vi "Third Restarts by Flow Sandbox (FPGA).vi"() -> ()   [LabVIEW 2019]
uses:
  <vilib>/eio/EIONode/EIONode.xnode
  <vilib>/rvi/eio/common/nirviEmuTemplateMethod_errors.vi
  <vilib>/rvi/FXPMathLib/FxpMul/XNode/nifxpmath_Multiplier.xnode
  <vilib>/rvi/FXPMathLib/sim/FxpSim.dll
  <vilib>/Platform/TimedLoop/XDataNode/wakeup.ctl
  <vilib>/Platform/TimedLoop/XDataNode/XDNodeRunTimeDep.lvlib
  <vilib>/Platform/TimedLoop/XDataNode/nitl_modes.ctl
  <vilib>/Platform/TimedLoop/XDataNode/timing_clust.ctl
  <vilib>/Platform/TimedLoop/XDataNode/XDataNode.xnode
  <vilib>/rvi/Analysis/measure/dc-rms/XNode/niFpgaDC-RMS.xnode
  <vilib>/rvi/DataTransferAndStorage/Container/XNode/niFpgaContainer.xnode
  <vilib>/rvi/FXPMathLib/FxpAdd/XNode/nifxpmath_Add.xnode
  <userlib>/_NI SPI IP/FPGA/Controllers/Public/Spi Master Inputs.ctl
  <vilib>/eio/EIOMethodNode/EIOMethodNode.xnode
  Controls/SPI Channels.ctl
  <vilib>/rvi/FIFO/Fifo_Resource/niFpgaFifoEmulationRefIn.vi
  <vilib>/rvi/interface/RandomDataEmulation/nirviRandomDataFpgaReadWriteTemplate.vi
  <vilib>/rvi/FXPMathLib/basic elements/FxpIntAccumulator/simVIs/DllFxpIntAccumulator_sub.vi
  <vilib>/rvi/FXPMathLib/basic elements/FxpIntAccumulator/XNode/nifxpmath_IntAccumulator.xnode
  <vilib>/rvi/FXPMathLib/FxpSqrt/XNode/nifxpmath_Sqrt.xnode
  <vilib>/rvi/Analysis/common/codeGenErrors/XNode/niFpgaXNodeCodeGenErrorHandle.vi
  <vilib>/rvi/FXPMathLib/FxpSqrt/simVIs/DllSqrtTemp_sub.vi
  <vilib>/fxp/LVFixedPointOverflowPolicyTypeDef.ctl
  <vilib>/rvi/FXPMathLib/FxpSqrt/subVIs/nifxpmath_Sqrt_SimConfig.ctl
  <vilib>/rvi/FXPMathLib/basic elements/FxpIntAccumulator/subVIs/nifxpmath_IntAccumulator_SimConfig.ctl
  <vilib>/rvi/FXPMathLib/FxpSub/XNode/nifxpmath_Sub.xnode
  <userlib>/_NI SPI IP/FPGA/Controllers/Public/Transfer Settings.ctl
panel:
  in  "Trigger":bool
  in  "Reset Restarts":bool
  in  "AI24-31 Data to Write":u64 format="%.0x"
  out "AI24-31":fxp<+/-,28,17>[](array[numeric])
  out "Read Data 2":u64 format="%.0x"
  in  "AI24-31 Settings":T1 {"Direction Change Bit" max=64 step=1; "Transfer Length (bits)" min=1 max=64 step=1}
  out "AI16-23":fxp<+/-,28,17>[](array[numeric])
  in  "AI16-23 Data to Write":u64 format="%.0x"
  out "Read Data":u64 format="%.0x"
  in  "AI16-23 Settings":T1 {"Direction Change Bit" max=64 step=1; "Transfer Length (bits)" min=1 max=64 step=1}
  in  "AO0":fxp<+/-,20,5>
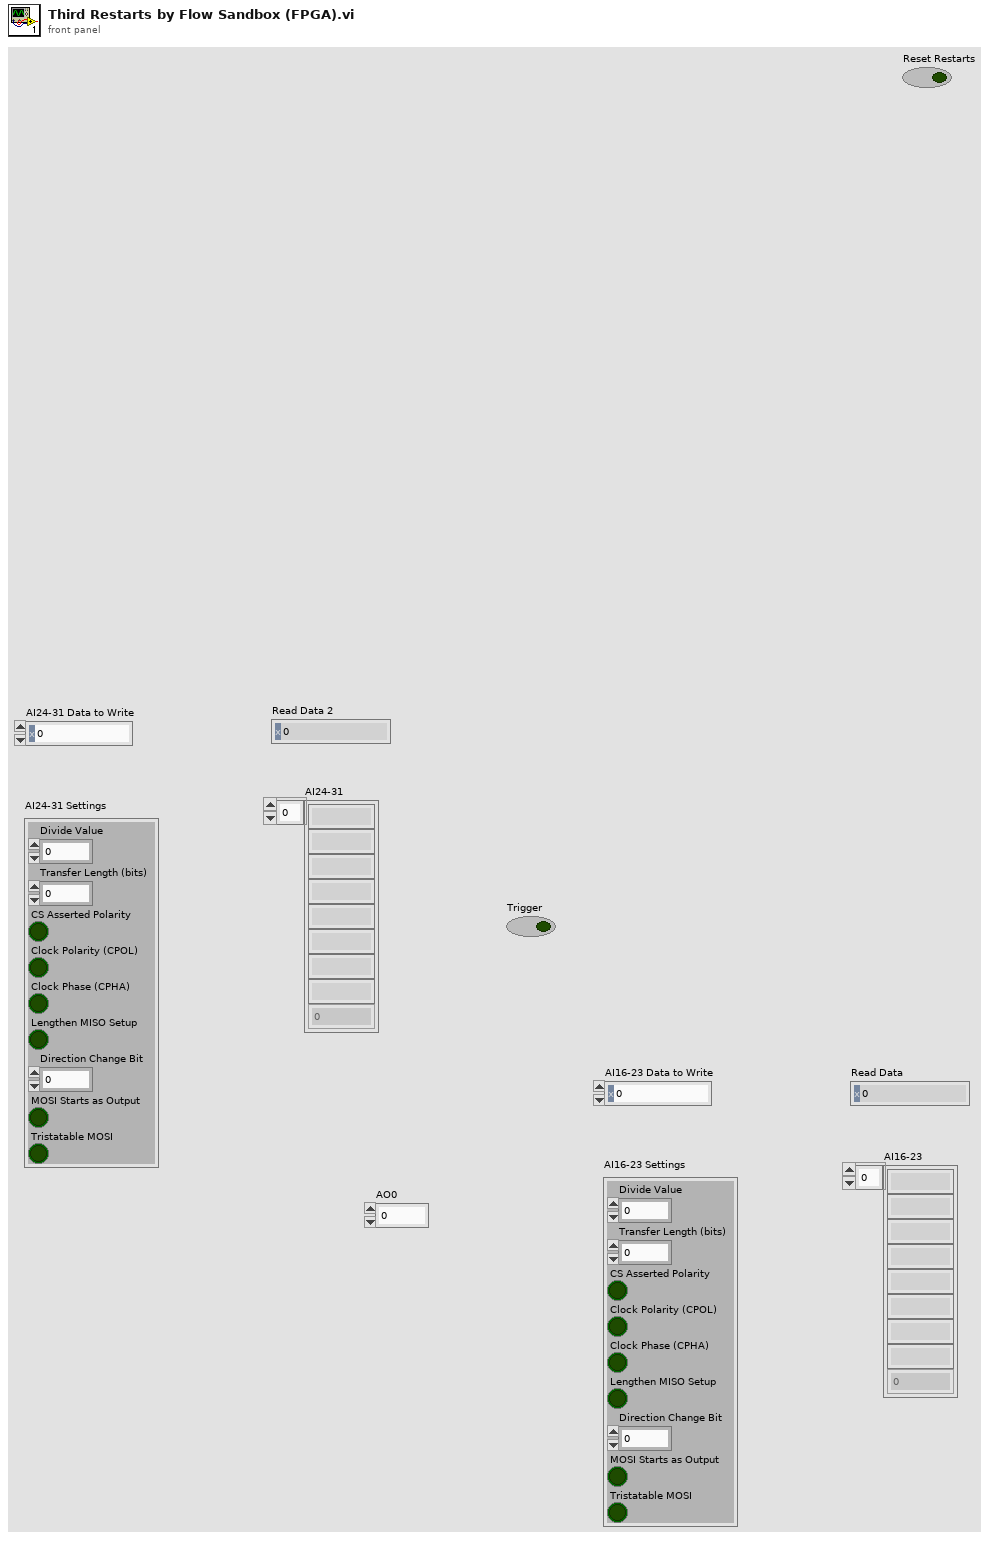
[diagram p1: front panel]
types:
  T1 = typedef "DIO SPI FPGA.lvlib/Transfer Settings.ctl" = cluster{"Divide Value":u8, "Transfer Length (bits)":u8, "CS Asserted Polarity":bool, "Clock Polarity (CPOL)":bool, "Clock Phase (CPHA)":bool, "Lengthen MISO Setup":bool, "Direction Change Bit":u8, "MOSI Starts as Output":bool, "Tristatable MOSI":bool}
  T2 = typedef "SPI Channels.ctl" = cluster{"CS":refnum<k21>, "CLK":refnum<k21>, "MOSI":refnum<k21>, "MISO":refnum<k21>}
  T3 = typedef "XDNodeRunTimeDep.lvlib/timing_clust.ctl" = cluster{"Expected End [f-1]":u64, "Actual End [f-1]":u64, "Finished Late? [f-1]":bool, "Expected End [i-1]":u64, "Actual End [i-1]":u64, "Finished Late? [i-1]":bool, "Expected Start [i]":u64, "Actual Start [i]":u64, "Expected Start [f]":u64, "Actual Start [f]":u64, "Source Name":string, "Structure Name":string, "Period":i64, "Deadline":i64, "Offset":i64, "Start":i64, "Priority":i32, "Timeout":i32, "Mode":T4, "Wakeup Reason":T5, "Error":errorcluster, "Source Type":string, "Secondary Source Type":string, "Global End Time":u64, "Global Start Time":u64, "Frame Duration":u64, "Iteration Duration":u64, "Assigned CPU":i32, "I/O Scan Engine Mode":u32}
  T4 = typedef "XDNodeRunTimeDep.lvlib/nitl_modes.ctl" = enum32{"No Change", "Process missed periods, maintain original phase", "Discard missed periods, maintain original phase", "Process missed periods, ignore original phase", "Discard missed periods, ignore original phase"}
  T5 = typedef "XDNodeRunTimeDep.lvlib/wakeup.ctl" = enum32{"Normal", "Aborted", "Asynchronous wakeup", "Timing source error", "Timed loop error", "Timeout"}
  T6 = typedef "DIO SPI FPGA.lvlib/Spi Master Inputs.ctl" = cluster{"MISO":bool}
  T7 = typedef "DIO SPI FPGA.lvlib/Spi Master Outputs.ctl" = cluster{"Chip Select":bool, "Clock":bool, "MOSI":bool, "MOSI OE":bool}
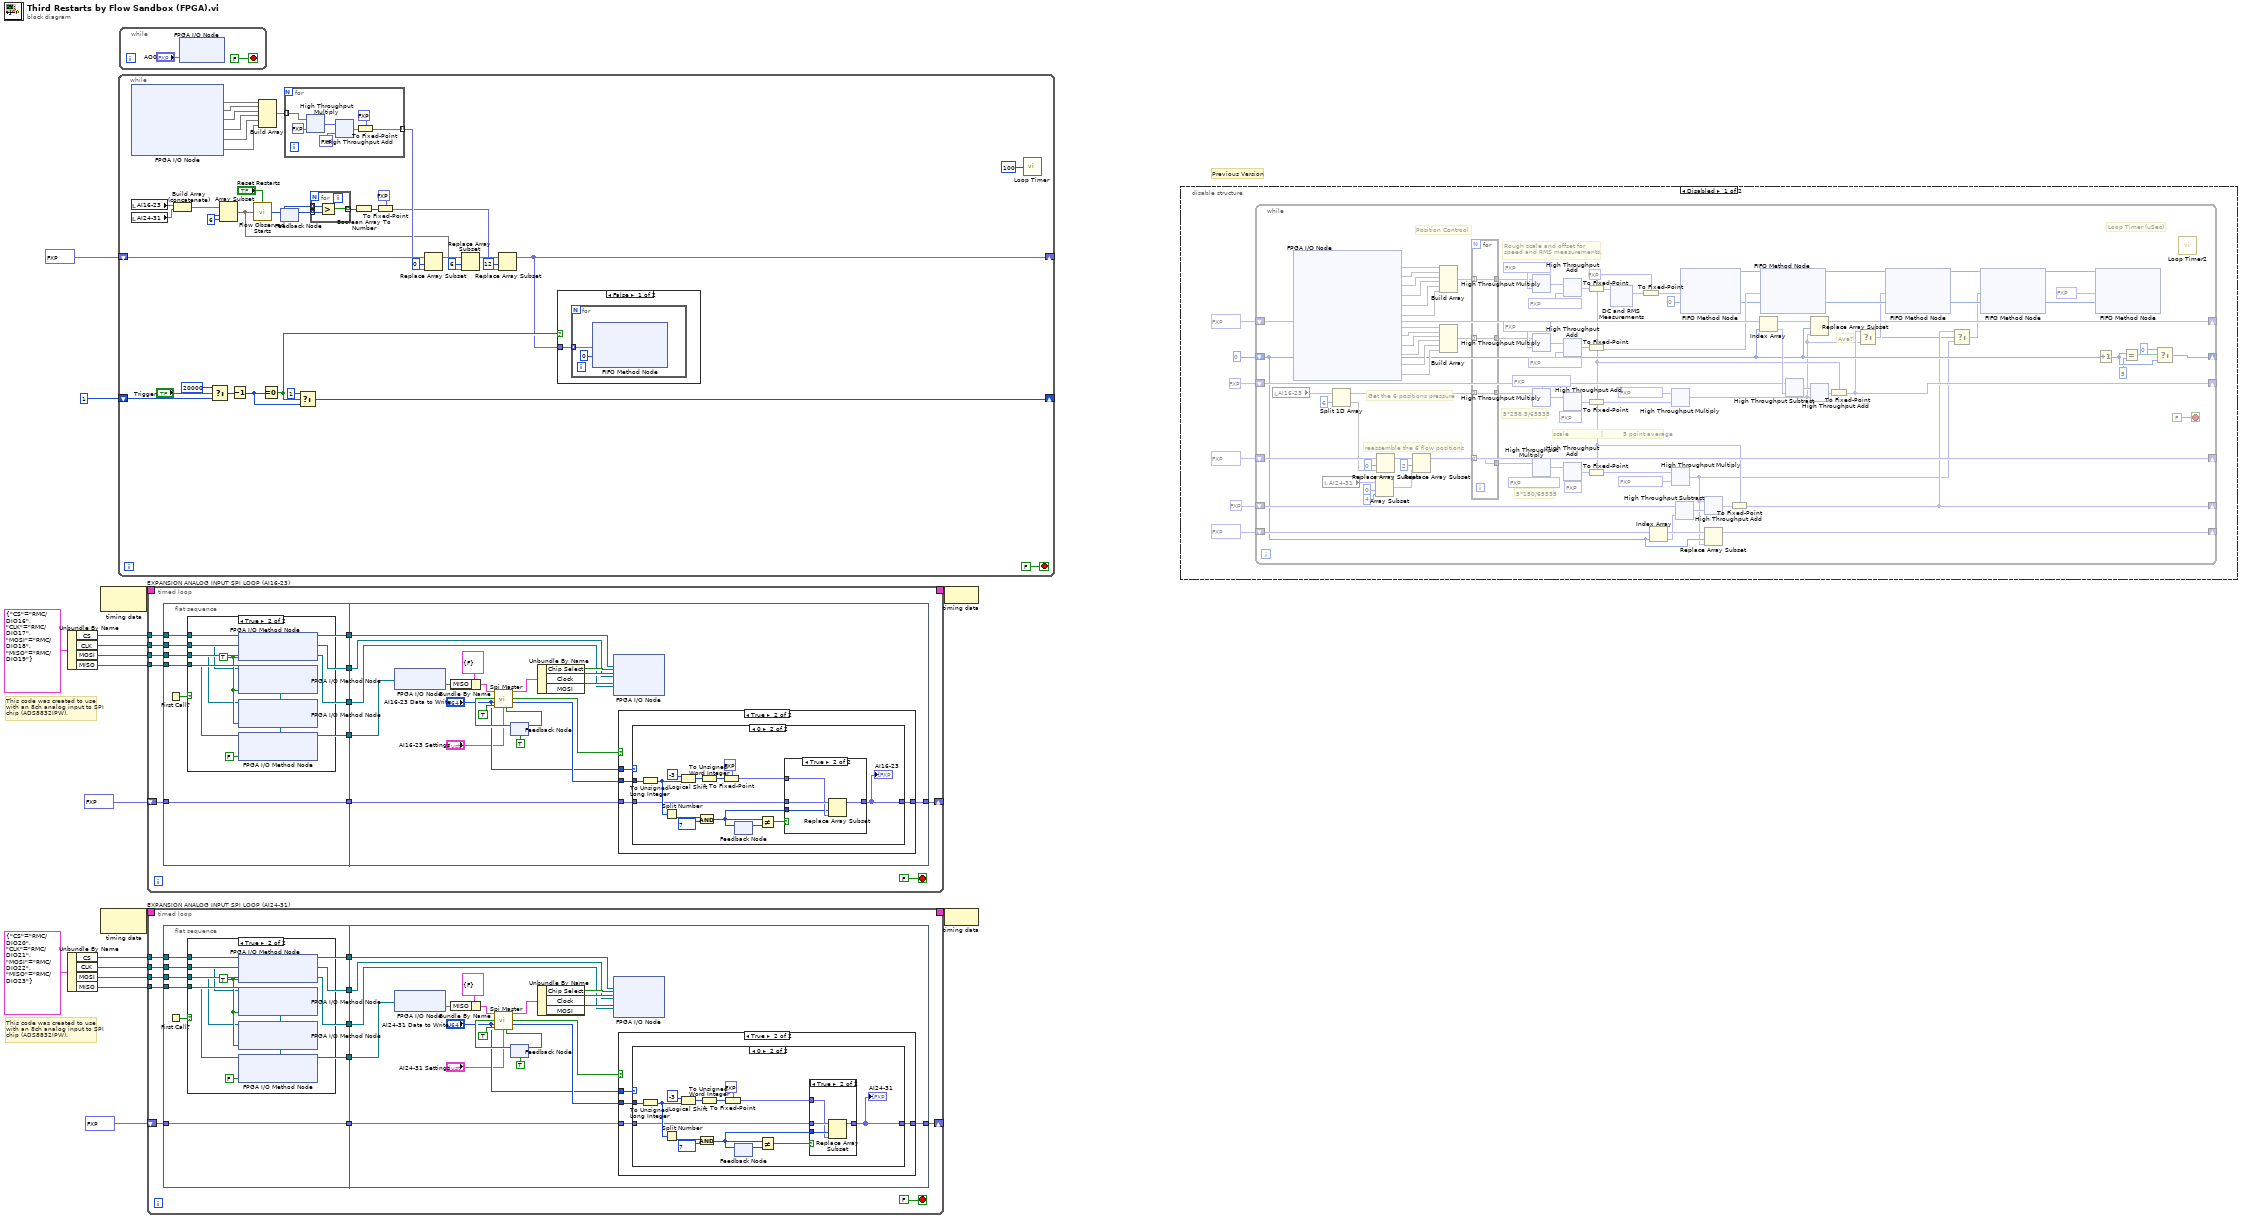
[diagram p0: block diagram]
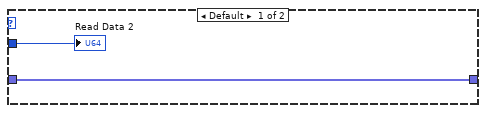
[diagram p6: hidden frame]
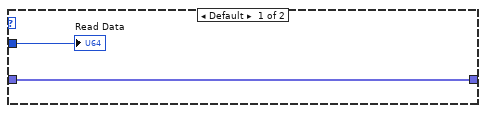
[diagram p10: hidden frame]
diagram:
  # "Previous Version"
  # "This code was created to use\nwith an 8ch analog input to SPI\nchip (ADS8832IPW)."
  # "This code was created to use\nwith an 8ch analog input to SPI\nchip (ADS8832IPW)."
  n1 = Unbundle By Name(T2 {"CS"="RMC/DIO16", "CLK"="RMC/DIO17", "MOSI"="RMC/DIO18", "MISO"="RMC/DIO19"} ("SPI Channels")) -> ("CS"=w12:refnum<k21>, "CLK"=w13:refnum<k21>, "MOSI"=w14:refnum<k21>, "MISO"=w15:refnum<k21>)
  n2 = Unbundle By Name(T2 {"CS"="RMC/DIO20", "CLK"="RMC/DIO21", "MOSI"="RMC/DIO22", "MISO"="RMC/DIO23"} ("SPI Channels")) -> ("CS"=w4:refnum<k21>, "CLK"=w5:refnum<k21>, "MOSI"=w6:refnum<k21>, "MISO"=w7:refnum<k21>)
  n3 = node-c288() -> (w18:T3)  [unwired: 1 in]
  n4 = node-c288() -> (w10:T3)  [unwired: 1 in]
  n5 = while {
    shift-right: [w36] -> _
    shift-left: i16 1 -> [w41]
    shift-right: [w19] -> _
    shift-left: fxp<+/-,28,17>[] [0.0, 0.0, 0.0, 0.0, 0.0, 0.0, 0.0, 0.0, 0.0, 0.0, 0.0, 0.0, 0.0] -> [w29]
    stop <- FALSE stop-if-true
    w44 = 6 ("length")
    n6 = xnode "FPGA I/O Node"() -> ("Speed_Current_1 (AI0)"=w46, "Speed_Current_2 (AI1)"=w51, "Speed_Current_3 (AI2)"=w50, "Speed_Current_4 (AI3)"=w49, "Speed_Current_5 (AI4)"=w48, "Speed_Current_6 (AI5)"=w47)  [unwired: 6 in, 6 out]
    n7 = local read "AI16-23"() -> (w54:fxp<+/-,28,17>[])
    n8 = local read "AI24-31"() -> (w55:fxp<+/-,28,17>[])
    n9 = Build Array (concatenate)(w54, w55) -> (w45:fxp<+/-,28,17>[])
    n10 = Select(t=i16 20000, s="Trigger", f=w41) -> (s? t:f=w39:i16)
    n11 = Array Subset(array=w45, index=w44, length=w44) -> (w25:fxp<+/-,28,17>[])
    n12 = Decrement(x=w39) -> (x-1=w38:i16)
    n13 = call "Flow Observed Starts.vi"("Reset Starts"="Reset Restarts", "Flows"=w25) -> ("Observed Starts"=w34:u32[])  [unwired: 13 in]
    n14 = Build Array(w46, w51, w50, w49, w48, w47) -> (w30:void[])
    n15 = Equal To 0?(x=w38) -> (x = 0?=w20:bool)
    n16 = feedback-in #1(w34) -> ()
    n17 = feedback #1(w34) -> (w35:u32[])
    n18 = for {
      tunnel: w30 -> [w60] mode=indexing
      tunnel: [w59] -> w26 mode=indexing
      n19 = xnode ("High Throughput Multiply")("x"=w60, "y"=fxp<+,5,5> 24.0 ("Current Scale")) -> ("x*y"=w63:fxp<+/-,29,10>)
      n20 = xnode ("High Throughput Add")("x"=w63, "y"=fxp<+/-,7,7> -60.0 ("Current Offset")) -> ("x+y"=w65:fxp<+/-,30,11>)
      n21 = To Fixed-Point(fixed-point type=fxp<+/-,28,17> 0.0 ("out"), number=w65) -> (fixed-point=w59:fxp<+/-,28,17>)
    }
    n22 = Select(t=i16 1, s=w20, f=w38) -> (s? t:f=w36:i16)
    n23 = for {
      tunnel: w35 -> [w67] mode=indexing
      tunnel: w34 -> [w68] mode=indexing
      tunnel: [w66] -> w33 mode=indexing
      n24 = Greater?(x=w68, y=w67) -> (0:w66:bool)
    }
    n25 = Boolean Array To Number(Boolean array=w33) -> (number=w31:u8)
    n26 = To Fixed-Point(fixed-point type=fxp<+/-,28,17> 0.0 ("out"), number=w31) -> (fixed-point=w24:fxp<+/-,28,17>)
    n27 = Replace Array Subset(array=w29, new element=w26, index=0) -> (w28:fxp<+/-,28,17>[])
    n28 = Replace Array Subset(array=w28, new element=w25, index=6) -> (w27:fxp<+/-,28,17>[])
    n29 = Replace Array Subset(array=w27, new element=w24, index=12) -> (w19:fxp<+/-,28,17>[])
    n30 = case shown="False" w20 {
      tunnel: w19 -> [w56 _]
      frame False {
        n31 = for {
          tunnel: w56 -> [w57] mode=indexing
          n32 = xnode ("FIFO Method Node")("Element"=w57, "Timeout"=0) -> ()  [unwired: 1 in, 2 out]
        }
      }
      frame True {
      }
    }
    n33 = call "Loop Timer"("Count(uSec)"=u32 100 ("Loop Timer (uSec)")) -> ()  [unwired: 1 out]
  }
  n34 = while {
    stop <- FALSE stop-if-true
    n35 = xnode "FPGA I/O Node"("AO0"="AO0") -> ()  [unwired: 2 in, 2 out]
  }
  n36 = timed-loop "EXPANSION ANALOG INPUT SPI LOOP (AI16-23)" {
    timing: w18 -> [_]
    timing-out: [_] -> w17
    shift-right: [w79] -> _
    shift-left: fxp<+/-,28,17>[] [0.0, 0.0, 0.0, 0.0, 0.0, 0.0, 0.0, 0.0] -> [w80]
    tunnel: w12 -> [w78]
    tunnel: w13 -> [w77]
    tunnel: w14 -> [w76]
    tunnel: w15 -> [w75]
    stop <- FALSE stop-if-true
    n37 = flat-sequence {
      tunnel: [w87] -> w81
      tunnel: w80 -> [w87]
      tunnel: w78 -> [w86]
      tunnel: w77 -> [w85]
      tunnel: w76 -> [w84]
      tunnel: w75 -> [w83]
      tunnel: [w86] -> w74
      tunnel: [w85] -> w73
      tunnel: [w84] -> w72
      tunnel: [w83] -> w71
      tunnel: w81 -> [w101]
      tunnel: [w100] -> w79
      tunnel: w74 -> [w99]
      tunnel: w73 -> [w98]
      tunnel: w72 -> [w97]
      tunnel: w71 -> [w96]
      frame #0 {
        n38 = First Call?() -> (First Call?: T/F=w88:bool)
        n39 = case shown="True" w88 {
          tunnel: w86 -> [_ w92]
          tunnel: w85 -> [_ w91]
          tunnel: w84 -> [_ w90]
          tunnel: w83 -> [_ w89]
          frame False {
          }
          frame True {
            w94 = TRUE ("Enable")
            n40 = xnode "FPGA I/O Method Node"("FPGA I/O In"=w92, "Enable"=w94) -> ()  [unwired: 1 out]
            n41 = xnode "FPGA I/O Method Node"("FPGA I/O In"=w91, "Enable"=w94) -> ()  [unwired: 1 out]
            n42 = xnode "FPGA I/O Method Node"("FPGA I/O In"=w90, "Enable"=w94) -> ()  [unwired: 1 out]
            n43 = xnode "FPGA I/O Method Node"("FPGA I/O In"=w89, "Enable"=FALSE) -> ()  [unwired: 1 out]
          }
        }
      }
      frame #1 {
        n44 = xnode "FPGA I/O Node"("FPGA I/O In"=w96) -> ("I/O Item"=w109)  [unwired: 1 out]
        n45 = Bundle By Name(cluster=T6 {"MISO"=FALSE} ("spi input"), "MISO"=w109) -> (w110:T6)
        n46 = feedback #2(TRUE ("read data valid")) -> (w106:bool)
        n47 = call <userlib>:"Spi Master.vi"("spi input"=w110, "start strobe"=w106, "data to write"="AI16-23 Data to Write", "MOSI output enable done"=TRUE, "spi transfer settings"="AI16-23 Settings") -> ("spi output"=w115:T7, "read data valid"=w102:bool, "read data"=w107:u64, "ready for input"=w103:bool)  [unwired: 7 in]
        n48 = feedback-in #2(w103) -> ()
        n49 = Unbundle By Name(w115) -> ("Chip Select"=w114:bool, "Clock"=w113:bool, "MOSI"=w112:bool)
        n50 = xnode "FPGA I/O Node"("I/O Item"=w114, "FPGA I/O In"=w99, "I/O Item"=w113, "FPGA I/O In"=w98, "I/O Item"=w112, "FPGA I/O In"=w97) -> ()  [unwired: 3 out]
        n51 = case shown="True" w102 {
          tunnel: w107 -> [_ w120]
          tunnel: "AI16-23 Data to Write" -> [_ w119]
          tunnel: w101 -> [w116 w118]
          tunnel: [w116 w117] -> w100
          frame False {
          }
          frame True {
            n52 = case shown="0" w119 {
              tunnel: w120 -> [w122 w136]
              tunnel: w118 -> [w121 w129]
              tunnel: [w121 w128] -> w117
              frame Default {
                "Read Data" <- w122
              }
              frame 0 {
                n53 = To Unsigned Long Integer(number=w136) -> (unsigned 32bit integer=w130:u32)
                n54 = Split Number(x=w130) -> (lo(x)=w134:u16)  [unwired: 1 out]
                n55 = Logical Shift(y=i16 -3, x=w130) -> (x << y=w131:u32)
                n56 = And(x=w134, y=u16 7) -> (x .and. y?=w126:u16)
                n57 = To Unsigned Word Integer(number=w131) -> (unsigned 16bit integer=w124:u16)
                n58 = To Fixed-Point(fixed-point type=fxp<+/-,28,17> 0.0 ("AI0"), number=w124) -> (fixed-point=w123:fxp<+/-,28,17>)
                n59 = feedback #3() -> (w135:u16)  [unwired: 1 in]
                n60 = feedback-in #3(w126) -> ()
                n61 = Not Equal?(x=w126, y=w135) -> (x != y?=w127:bool)
                n62 = case shown="True" w127 {
                  tunnel: w129 -> [w137 w141]
                  tunnel: [w137 w140] -> w128
                  tunnel: w126 -> [_ w138]
                  tunnel: w123 -> [_ w139]
                  frame False {
                  }
                  frame True {
                    n63 = Replace Array Subset(array=w141, new element=w139, index=w138) -> (w140:fxp<+/-,28,17>[])
                  }
                }
                "AI16-23" <- w128
              }
            }
          }
        }
      }
    }
  }
  n64 = timed-loop "EXPANSION ANALOG INPUT SPI LOOP (AI24-31)" {
    timing: w10 -> [_]
    timing-out: [_] -> w9
    shift-right: [w152] -> _
    shift-left: fxp<+/-,28,17>[] [0.0, 0.0, 0.0, 0.0, 0.0, 0.0, 0.0, 0.0] -> [w153]
    tunnel: w4 -> [w151]
    tunnel: w5 -> [w150]
    tunnel: w6 -> [w149]
    tunnel: w7 -> [w148]
    stop <- FALSE stop-if-true
    n65 = flat-sequence {
      tunnel: [w160] -> w154
      tunnel: w153 -> [w160]
      tunnel: w151 -> [w159]
      tunnel: w150 -> [w158]
      tunnel: w149 -> [w157]
      tunnel: w148 -> [w156]
      tunnel: [w159] -> w147
      tunnel: [w158] -> w146
      tunnel: [w157] -> w145
      tunnel: [w156] -> w144
      tunnel: w154 -> [w174]
      tunnel: [w173] -> w152
      tunnel: w147 -> [w172]
      tunnel: w146 -> [w171]
      tunnel: w145 -> [w170]
      tunnel: w144 -> [w169]
      frame #0 {
        n66 = First Call?() -> (First Call?: T/F=w161:bool)
        n67 = case shown="True" w161 {
          tunnel: w159 -> [_ w165]
          tunnel: w158 -> [_ w164]
          tunnel: w157 -> [_ w163]
          tunnel: w156 -> [_ w162]
          frame False {
          }
          frame True {
            w167 = TRUE ("Enable")
            n68 = xnode "FPGA I/O Method Node"("FPGA I/O In"=w165, "Enable"=w167) -> ()  [unwired: 1 out]
            n69 = xnode "FPGA I/O Method Node"("FPGA I/O In"=w164, "Enable"=w167) -> ()  [unwired: 1 out]
            n70 = xnode "FPGA I/O Method Node"("FPGA I/O In"=w163, "Enable"=w167) -> ()  [unwired: 1 out]
            n71 = xnode "FPGA I/O Method Node"("FPGA I/O In"=w162, "Enable"=FALSE) -> ()  [unwired: 1 out]
          }
        }
      }
      frame #1 {
        n72 = xnode "FPGA I/O Node"("FPGA I/O In"=w169) -> ("I/O Item"=w182)  [unwired: 1 out]
        n73 = Bundle By Name(cluster=T6 {"MISO"=FALSE} ("spi input"), "MISO"=w182) -> (w183:T6)
        n74 = feedback #4(TRUE ("read data valid")) -> (w179:bool)
        n75 = call <userlib>:"Spi Master.vi"("spi input"=w183, "start strobe"=w179, "data to write"="AI24-31 Data to Write", "MOSI output enable done"=TRUE, "spi transfer settings"="AI24-31 Settings") -> ("spi output"=w188:T7, "read data valid"=w175:bool, "read data"=w180:u64, "ready for input"=w176:bool)  [unwired: 7 in]
        n76 = feedback-in #4(w176) -> ()
        n77 = Unbundle By Name(w188) -> ("Chip Select"=w187:bool, "Clock"=w186:bool, "MOSI"=w185:bool)
        n78 = xnode "FPGA I/O Node"("I/O Item"=w187, "FPGA I/O In"=w172, "I/O Item"=w186, "FPGA I/O In"=w171, "I/O Item"=w185, "FPGA I/O In"=w170) -> ()  [unwired: 3 out]
        n79 = case shown="True" w175 {
          tunnel: w180 -> [_ w193]
          tunnel: "AI24-31 Data to Write" -> [_ w192]
          tunnel: w174 -> [w189 w191]
          tunnel: [w189 w190] -> w173
          frame False {
          }
          frame True {
            n80 = case shown="0" w192 {
              tunnel: w193 -> [w195 w209]
              tunnel: w191 -> [w194 w202]
              tunnel: [w194 w201] -> w190
              frame Default {
                "Read Data 2" <- w195
              }
              frame 0 {
                n81 = To Unsigned Long Integer(number=w209) -> (unsigned 32bit integer=w203:u32)
                n82 = Split Number(x=w203) -> (lo(x)=w207:u16)  [unwired: 1 out]
                n83 = Logical Shift(y=i16 -3, x=w203) -> (x << y=w204:u32)
                n84 = And(x=w207, y=u16 7) -> (x .and. y?=w199:u16)
                n85 = To Unsigned Word Integer(number=w204) -> (unsigned 16bit integer=w197:u16)
                n86 = To Fixed-Point(fixed-point type=fxp<+/-,28,17> 0.0 ("AI0"), number=w197) -> (fixed-point=w196:fxp<+/-,28,17>)
                n87 = feedback #5() -> (w208:u16)  [unwired: 1 in]
                n88 = feedback-in #5(w199) -> ()
                n89 = Not Equal?(x=w199, y=w208) -> (x != y?=w200:bool)
                n90 = case shown="True" w200 {
                  tunnel: w202 -> [w210 w214]
                  tunnel: [w210 w213] -> w201
                  tunnel: w199 -> [_ w212]
                  tunnel: w196 -> [_ w211]
                  frame False {
                  }
                  frame True {
                    n91 = Replace Array Subset(array=w214, new element=w211, index=w212) -> (w213:fxp<+/-,28,17>[])
                  }
                }
                "AI24-31" <- w201
              }
            }
          }
        }
      }
    }
  }
  n92 = node-c288(w17) -> ()
  n93 = node-c288(w9) -> ()
  n94 = disable-structure shown="Disabled" {
    frame Disabled {
      n95 = while {
        shift-right: [w275] -> _
        shift-left: fxp<+/-,28,17>[] [0.0, 0.0, 0.0, 0.0, 0.0] -> [w269]
        shift-right: [w270] -> _
        shift-left: 0 -> [w235]
        shift-right: [w229] -> _
        shift-left: fxp<+/-,28,17> 0.0 -> [w264]
        shift-right: [w250] -> _
        shift-left: fxp<+/-,28,17>[] [0.0, 0.0, 0.0, 0.0, 0.0, 0.0] -> [w259]
        shift-right: [w236] -> _
        shift-left: fxp<+/-,28,17>[] [0.0, 0.0, 0.0, 0.0, 0.0] -> [w240]
        shift-right: [w227] -> _
        shift-left: fxp<+/-,28,17> 0.0 ("AI0") -> [w238]
        stop <- FALSE stop-if-true
        w230 = 0 ("Timeout")
        w232 = fxp<+/-,28,17> 0.0 ("out")
        # "Loop Timer (uSec)"
        # "Ave?"
        # "Position Controol"
        # "scale                |          5 point average"
        # "5*150/65535"
        # "reassemble the 6 flow positions"
        # "Get the 6 positions pressure"
        # "5*258.5/65535"
        # "Rough scale and offset for\nspeed and RMS measurements."
        n96 = local read "AI16-23"() -> (w262:fxp<+/-,28,17>[])
        n97 = xnode "FPGA I/O Node"() -> ("Speed_Current_1 (AI0)"=w306, "Speed_Current_2 (AI1)"=w312, "Speed_Current_3 (AI2)"=w311, "Speed_Current_4 (AI3)"=w310, "Speed_Current_5 (AI4)"=w309, "Speed_Current_6 (AI5)"=w308, "Controller_Current_1 (AI6)"=w296, "Controller_Current_2 (AI7)"=w295, "Controller_Current_3 (AI8)"=w294, "Controller_Current_4 (AI9)"=w293, "Controller_Current_5 (AI10)"=w292, "Controller_Current_6 (AI11)"=w291)  [unwired: 12 in, 12 out]
        n98 = local read "AI24-31"() -> (w257:fxp<+/-,28,17>[])
        n99 = Split 1D Array(array=w262, index=6) -> (first subarray=w260:fxp<+/-,28,17>[], second subarray=w251:fxp<+/-,28,17>[])
        n100 = Array Subset(array=w257, index=0, length=4) -> (w255:fxp<+/-,28,17>[])
        n101 = Replace Array Subset(array=w259, new element=w251, index=0) -> (w258:fxp<+/-,28,17>[])
        n102 = Replace Array Subset(array=w258, new element=w255, index=2) -> (w250:fxp<+/-,28,17>[])
        n103 = Build Array(w306, w312, w311, w310, w309, w308) -> (w304:void[])
        n104 = Build Array(w296, w295, w294, w293, w292, w291) -> (w305:void[])
        n105 = for {
          N: [_] -> w297
          tunnel: w305 -> [w423] mode=indexing
          tunnel: w260 -> [w422] mode=indexing
          tunnel: w304 -> [w424] mode=indexing
          tunnel: [w424] -> w298
          tunnel: [w423] -> w287
          tunnel: [w422] -> w282
          tunnel: w250 -> [w421] mode=indexing
          tunnel: [w421] -> w246
        }
        n106 = xnode ("High Throughput Multiply")("x"=w298, "y"=fxp<+,16,5> 24.0380859375 ("Current Scale")) -> ("x*y"=w303:fxp<+/-,40,10>)
        n107 = xnode ("High Throughput Multiply")("x"=w287, "y"=fxp<+,16,5> 24.0380859375 ("Current Scale")) -> ("x*y"=w290:fxp<+/-,40,10>)
        n108 = xnode ("High Throughput Multiply")("x"=w282, "y"=fxp<+,20,6> 0.01971435546875 ("Current Scale")) -> ("x*y"=w283:fxp<+/-,48,23>)
        n109 = xnode ("High Throughput Multiply")("x"=w246, "y"=fxp<+,20,6> 0.011474609375) -> ("x*y"=w245:fxp<+/-,48,23>)
        n110 = xnode ("High Throughput Add")("x"=w303, "y"=fxp<+/-,18,7> -60.09521484375 ("Current Offset")) -> ("x+y"=w299:fxp<+/-,41,11>)
        n111 = xnode ("High Throughput Add")("x"=w290, "y"=fxp<+/-,18,7> -60.09521484375 ("Current Offset")) -> ("x+y"=w286:fxp<+/-,41,11>)
        n112 = xnode ("High Throughput Add")("x"=w283, "y"=fxp<+/-,21,10> -258.5 ("Current Offset")) -> ("x+y"=w281:fxp<+/-,49,24>)
        n113 = xnode ("High Throughput Add")("x"=w245, "y"=fxp<+/-,21,10> -150.0 ("Current Offset")) -> ("x+y"=w243:fxp<+/-,49,24>)
        n114 = To Fixed-Point(fixed-point type=w232, number=w299) -> (fixed-point=w300:fxp<+/-,28,17>)
        n115 = To Fixed-Point(fixed-point type=w232, number=w286) -> (fixed-point=w263:fxp<+/-,28,17>)
        n116 = To Fixed-Point(fixed-point type=w232, number=w281) -> (fixed-point=w233:fxp<+/-,28,17>)
        n117 = To Fixed-Point(fixed-point type=w232, number=w243) -> (fixed-point=w241:fxp<+/-,28,17>)
        n118 = xnode ("DC and RMS Measurements")("input data"=w300) -> ("RMS"=w277:fxp<+,28,17>)  [unwired: 1 in, 1 out]
        n119 = To Fixed-Point(fixed-point type=w232, number=w277) -> (fixed-point=w276:fxp<+/-,28,17>)
        n120 = Index Array(array=w240, index=w235) -> (element=w239:fxp<+/-,28,17>)
        n121 = xnode ("High Throughput Multiply")("x"=fxp<+,16,5> 0.2001953125 ("y"), "y"=w233) -> ("x*y"=w228:fxp<+/-,28,17>)
        n122 = xnode ("High Throughput Multiply")("x"=w241, "y"=fxp<+,16,5> 0.2001953125) -> ("x*y"=w226:fxp<+/-,28,17>)
        n123 = xnode "High Throughput Subtract"("x"=w238, "y"=w239) -> ("x-y"=w231:fxp<+/-,29,18>)
        n124 = xnode ("FIFO Method Node")("Element"=w276, "Timeout"=w230) -> ("FIFO Out"=w280:refnum<k21>)  [unwired: 1 in, 1 out]
        n125 = xnode ("High Throughput Add")("x"=w226, "y"=w231) -> ("x+y"=w237:fxp<+/-,30,19>)
        n126 = Replace Array Subset(array=w240, new element=w226, index=w235) -> (w236:fxp<+/-,28,17>[])
        n127 = To Fixed-Point(fixed-point type=w232, number=w237) -> (fixed-point=w227:fxp<+/-,28,17>)
        n128 = Index Array(array=w269, index=w235) -> (element=w268:fxp<+/-,28,17>)
        n129 = xnode ("FIFO Method Node")("Element"=w263, "Timeout"=w230, "FIFO In"=w280) -> ("FIFO Out"=w279:refnum<k21>)  [unwired: 1 out]
        n130 = xnode "High Throughput Subtract"("x"=w264, "y"=w268) -> ("x-y"=w267:fxp<+/-,29,18>)
        n131 = Replace Array Subset(array=w269, new element=w228, index=w235) -> (w275:fxp<+/-,28,17>[])
        n132 = xnode ("High Throughput Add")("x"=w267, "y"=w228) -> ("x+y"=w265:fxp<+/-,30,19>)
        n133 = To Fixed-Point(fixed-point type=w232, number=w265) -> (fixed-point=w229:fxp<+/-,28,17>)
        n134 = Select(t=w229, f=w228) -> (s=w223:bool, s? t:f=w224:fxp<+/-,28,17>)
        n135 = xnode ("FIFO Method Node")("Element"=w224, "Timeout"=w230, "FIFO In"=w279) -> ("FIFO Out"=w249:refnum<k21>)  [unwired: 1 out]
        n136 = Select(t=w227, s=w223, f=w226) -> (s? t:f=w225:fxp<+/-,28,17>)
        n137 = xnode ("FIFO Method Node")("Element"=w225, "Timeout"=w230, "FIFO In"=w249) -> ("FIFO Out"=w248:refnum<k21>)  [unwired: 1 out]
        n138 = xnode ("FIFO Method Node")("Element"=fxp<+/-,28,17> -9999.0 ("AI0"), "Timeout"=w230, "FIFO In"=w248) -> ()  [unwired: 2 out]
        n139 = Increment(x=w235) -> (x+1=w273:i32)
        n140 = Equal?(x=w273, y=5) -> (x = y?=w274:bool)
        n141 = Select(t=0, s=w274, f=w273) -> (s? t:f=w270:i32)
        n142 = call "Loop Timer2"() -> ("Count(uSec)"=w266:u32)  [unwired: 1 out]
      }
    }
    frame Enabled {
    }
  }
